vi "数据插入.vi"(5 "数据标记表":string(combo)="N", 7 "测量模式":string(combo), 8 "error in (no error)":errorcluster caption="错误输入（无错误）", 10 "data in":T1={"因子编码"="", "单位"="", "标样参考值"=0.0, "水样数据时间"=timestamp(0 s since 1904-01-01), "水样实测值"=0.0, "水样数据标识"="N", "探头温度"=0.0}, 11 "table输入":string(combo)) -> (0 "error out":errorcluster caption="错误输出")   [LabVIEW 2016, in "斯坦道多参数.lvlib"]
uses:
  <vilib>/addons/database/Connection.llb/DB Tools Open Connec (String).vi
  <vilib>/addons/database/NI_Database_API.lvlib
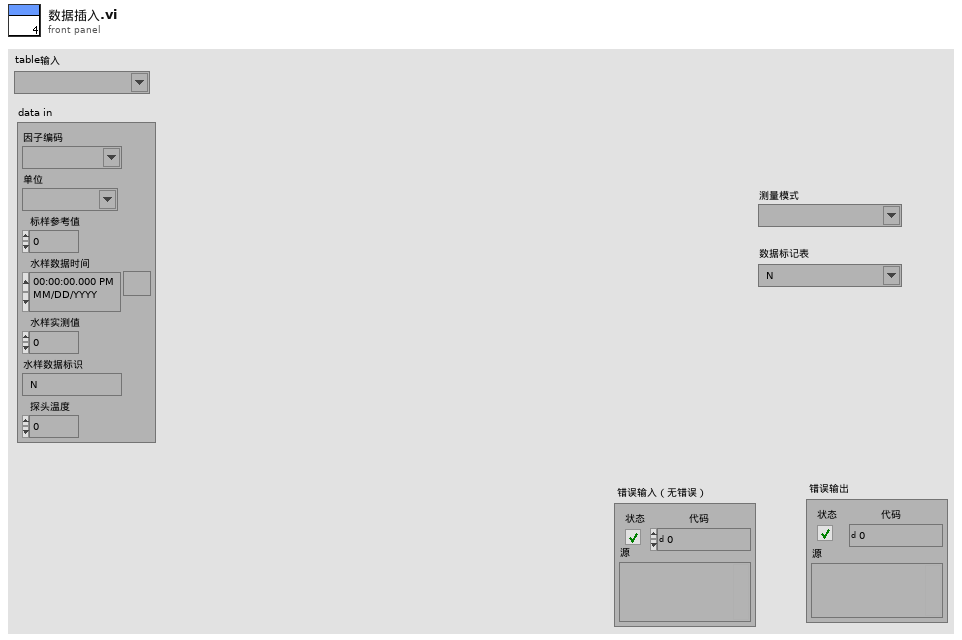
[diagram p1: front panel]
types:
  T1 = cluster{"因子编码":string, "单位":string, "标样参考值":sgl, "水样数据时间":timestamp, "水样实测值":sgl, "水样数据标识":string, "探头温度":sgl}
  T2 = cluster{"时间标识":timestamp, "测量模式":string, "数据类型":string, "监测值":sgl, "单位":string, "数据标识":string, "因子编码":string, "标样参考值":sgl, "探头温度":sgl}
  T3 = typedef "NI_Database_API.lvlib/Conn ObjectReference.ctl" = refnum<k1>
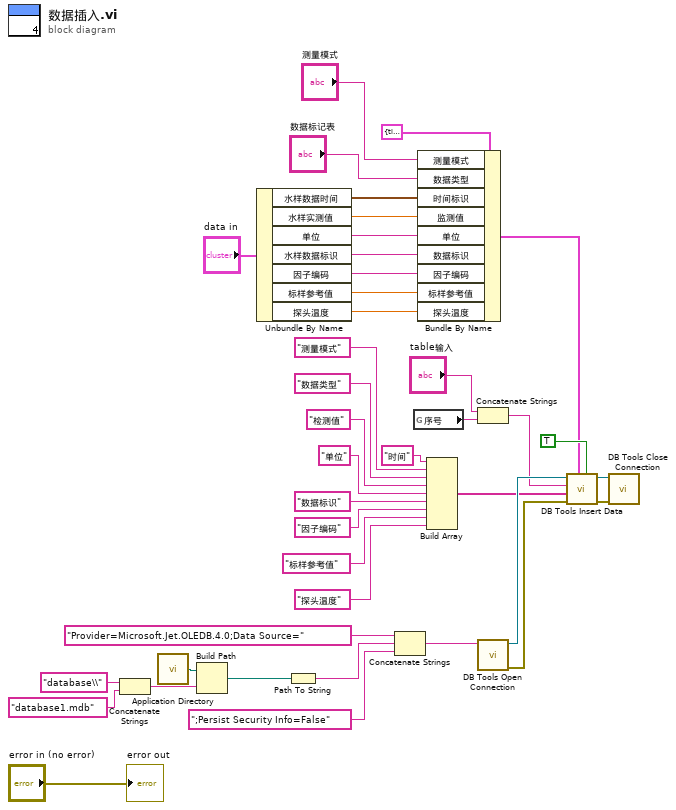
[diagram p0: block diagram]
diagram:
  n1 = Concatenate Strings("database\\" ("condition"), "database1.mdb" ("字符串")) -> (w15:string)
  n2 = call <vilib>:"Application Directory.vi"() -> ("Application Directory"=w3:path)
  n3 = Build Path(base path=w3, name or relative path=w15) -> (appended path=w20:path)
  n4 = Unbundle By Name("data in") -> ("水样数据时间"=w35:timestamp, "水样实测值"=w34:sgl, "单位"=w30:string, "水样数据标识"=w33:string, "因子编码"=w29:string, "标样参考值"=w31:sgl, "探头温度"=w9:sgl)
  n5 = Path To String(path=w20) -> (string=w19:string)
  n6 = Concatenate Strings("Provider=Microsoft.Jet.OLEDB.4.0;Data Source=" ("condition"), w19, ";Persist Security Info=False" ("condition")) -> (w17:string)
  n7 = global read "多参数全局变量.vi" "序号"() -> (w1:string)
  n8 = Bundle By Name(cluster=T2 {"时间标识"=timestamp(0 s since 1904-01-01), "测量模式"="", "数据类型"="", "监测值"=0.0, "单位"="", "数据标识"="", "因子编码"="", "标样参考值"=0.0, "探头温度"=0.0} ("data输出"), "测量模式"="测量模式", "数据类型"="数据标记表", "时间标识"=w35, "监测值"=w34, "单位"=w30, "数据标识"=w33, "因子编码"=w29, "标样参考值"=w31, "探头温度"=w9) -> (w11:T2)
  n9 = Build Array("时间", "测量模式", "数据类型", "检测值", "单位", "数据标识", "因子编码", "标样参考值", "探头温度") -> (w12:string[])
  n10 = Concatenate Strings("table输入", w1) -> (w2:string)
  n11 = call-poly <vilib>:"DB Tools Open Connection.vi"("connection information"=w17) -> ("error out"=w13:errorcluster, "connection reference"=w14:T3)  [unwired: 7 in]
  n12 = call <vilib>:"DB Tools Insert Data.vi"("create table? (F)"=TRUE, "data"=w11, "error in (no error)"=w13, "columns"=w12, "table"=w2, "connection reference"=w14) -> ("error out"=w23:errorcluster, "connection reference out"=w24:T3)  [unwired: 4 in]
  n13 = call <vilib>:"DB Tools Close Connection.vi"("error in (no error)"=w23, "connection reference"=w24) -> ()  [unwired: 5 in, 1 out]
  "error out" <- "error in (no error)"
